vi "State machine control.vi"() -> ()   [LabVIEW 2018]
panel:
  in  "Speed":dbl
  in  "Direction":T1(ring)
  in  "stop":bool
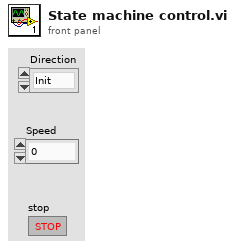
[diagram p1: front panel]
types:
  T1 = enum16{"Init", "Front Back", "Left Right", "Rotate", "Latch"}
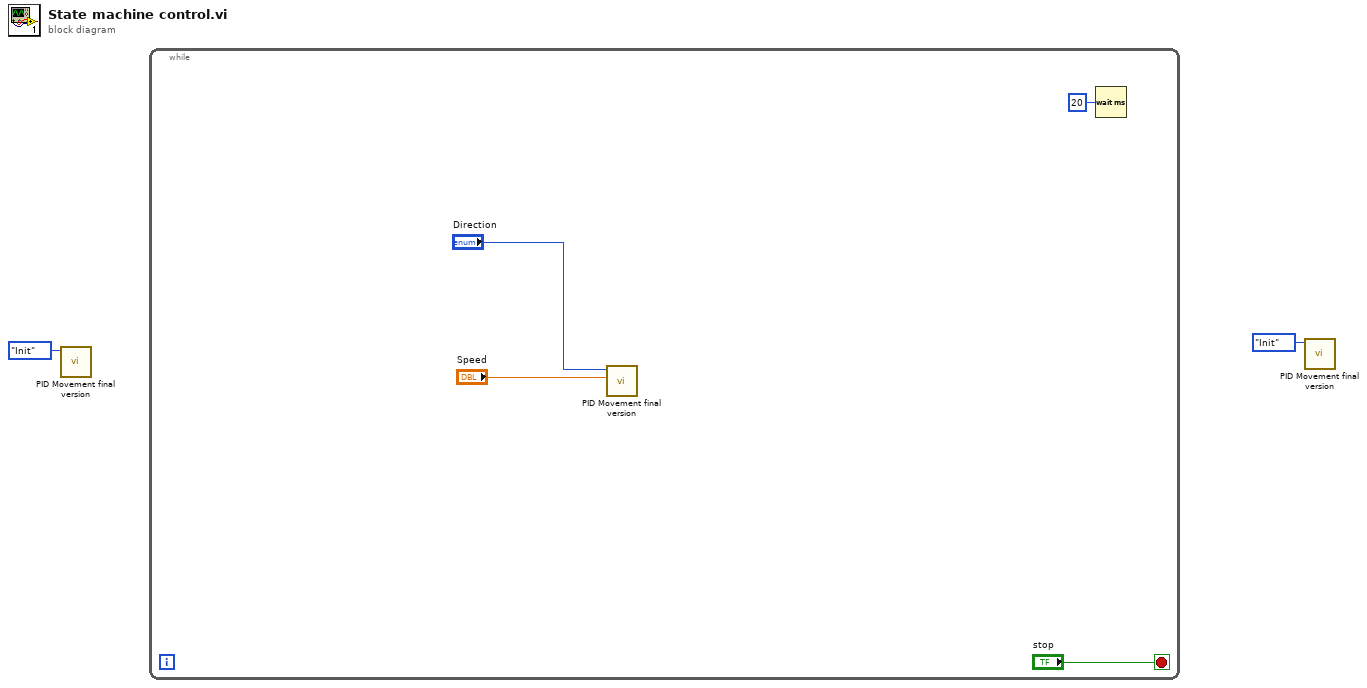
[diagram p0: block diagram]
diagram:
  n1 = call "PID Movement final version.vi"("Direction"=T1."Init") -> ()  [unwired: 3 in, 2 out]
  n2 = while {
    stop <- "stop" stop-if-true
    n3 = call "PID Movement final version.vi"("Speed"="Speed", "Direction"="Direction") -> ()  [unwired: 2 in, 2 out]
    n4 = Wait (ms)(milliseconds to wait=u32 20) -> ()  [unwired: 1 out]
  }
  n5 = call "PID Movement final version.vi"("Direction"=T1."Init") -> ()  [unwired: 3 in, 2 out]
